vi "new.vi"(8 "error in":errorcluster, 11 "Websocket console plugin in":refnum<class "Websocket console plugin.lvclass">) -> (0 "error out":errorcluster, 3 "Websocket console plugin out":refnum<class "Websocket console plugin.lvclass">)   [LabVIEW 2013, in "Websocket console plugin.lvclass"]
uses:
  Websocket console plugin.lvclass
  Websocket console plugin.lvclass/Websocket console plugin.ctl
  console UI.vi
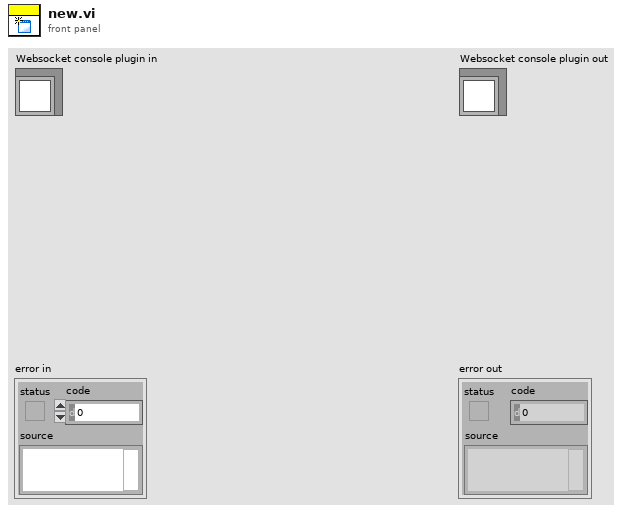
[diagram p1: front panel]
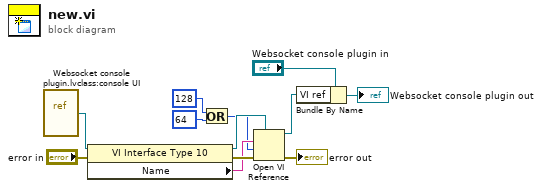
[diagram p0: block diagram]
diagram:
  n1 = vi-ref "Websocket console plugin.lvclass:console UI.vi"() -> (w11:refnum<vi>)
  n2 = property class="VI Interface Type 10"(reference=w11, error in="error in") -> (reference out=w8:refnum<vi>, error out=w10:errorcluster, "Name"=w9:string)
  n3 = Or(x=128 ("options"), y=64 ("options")) -> (x .or. y?=w7:i32)
  n4 = Open VI Reference(type specifier VI Refnum (for type only)=w8, vi path=w9, options=w7, error in (no error)=w10) -> (vi reference=w1:refnum<vi>, error out=→"error out":errorcluster)  [unwired: 2 in]
  n5 = Bundle By Name(cluster="Websocket console plugin in", "VI ref"=w1) -> (→"Websocket console plugin out":refnum<class "Websocket console plugin.lvclass">)
